vi "Add Target Listener.vi"(8 "error in":errorcluster, 11 "queue out":T1) -> (0 "error out":errorcluster)   [LabVIEW 2016, in "Vision Server.lvclass"]
uses:
  Vision Server.lvclass
  typedef/Target Listener Queue.ctl
  typedef/Target Message JSON.ctl
  typedef/Target Vector.ctl
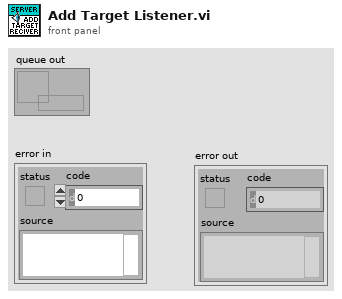
[diagram p1: front panel]
types:
  T1 = typedef "Vision Server.lvclass/Target Listener Queue.ctl" = refnum<queue>
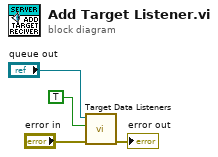
[diagram p0: block diagram]
diagram:
  n1 = call "Target Data Listeners.vi"("error in"="error in", "set? (F)"=TRUE, "Listener"="queue out") -> ("error out"=→"error out":errorcluster)  [unwired: 7 in, 1 out]
